vi "加计数器.vi"(8 "error in":errorcluster, 9 "preset value":u32=10, 10 "reset":bool, 11 "count up":bool) -> (0 "error out":errorcluster, 1 "counter value":u32, 3 "done":bool)   [LabVIEW 2013]
uses:
  <vilib>/ptbypt/NI_PtbyPt.lvlib
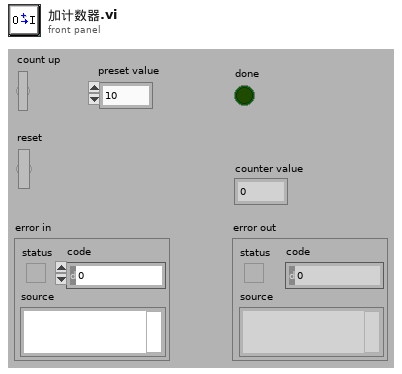
[diagram p1: front panel]
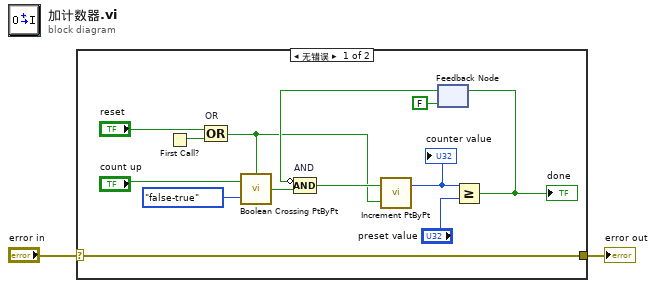
[diagram p0: block diagram]
diagram:
  n1 = case shown="无错误" "error in" {
    selector: "error in" -> [w15 w16]
    tunnel: [w15 w16] -> w2
    frame No Error {
      n2 = First Call?() -> (First Call?: T/F=w11:bool)
      n3 = Compound Arithmetic op=OR "OR"("reset", w11) -> (w4:bool)
      n4 = call <vilib>:"Boolean Crossing PtByPt.vi"("initialize"=w4, "direction"=enum16{"either", "false-true", "true-false"}."false-true", "input"="count up") -> ("crossing"=w5:bool)
      n5 = feedback #1(FALSE) -> (w6:bool)
      n6 = Compound Arithmetic op=AND "AND"(invert w6, w5) -> (w8:bool)
      n7 = call <vilib>:"Increment PtByPt.vi"("initialize"=w4, "activate"=w8) -> ("counter"=w9:u32)  [unwired: 1 out]
      "counter value" <- w9
      n8 = Greater Or Equal?(x=w9, y="preset value") -> (x >= y?=w7:bool)
      "done" <- w7
      n9 = feedback-in #1(w7) -> ()
    }
    frame Error {
    }
  }
  "error out" <- w2
